vi "Main.vi"(8 "error in":errorcluster, 11 "gRPC Read in":refnum<class "gRPC Read.lvclass">) -> (0 "error out":errorcluster, 3 "gRPC Read out":refnum<class "gRPC Read.lvclass">)   [LabVIEW 2019, in "gRPC Server (scope.proto).lvlib" / "gRPC Read.lvclass"]
doc: "The <b>Queued Message Handler</b> of the Worker that owns this VI."
uses:
  gRPC Read.lvclass
  Initialization Data.ctl
  Response Cases.ctl
  <vilib>/addons/_Workers/Library/Case Label.ctl
  <vilib>/gRPC/LabVIEW gRPC Library/Shared/grpcId.ctl
  gRPC Read.lvclass/gRPC Read.ctl
  rql_Read Incoming Data from Client.ctl
  Generated_server/RPC Messages/w4lvgrpc_ToServer_payload/w4lvgrpc_ToServer_payload.lvclass/w4lvgrpc_ToServer_payload.ctl
  Generated_server/RPC Messages/Get w4lvgrpc_ToServer.vi
  Generated_server/RPC Messages/Get w4lvgrpc_ToServer.vi/2ed25e12-861d-4677-8ead-ace2906b2041.vi
  Generated_server/RPC Messages/FlatToRichw4lvgrpc_ToServer.vi
  <vilib>/gRPC/LabVIEW gRPC Library/Shared/TranslateGrpcError.vi
  Generated_server/RPC Messages/w4lvgrpc_ToServer_payload/Setmsg_1.vi
  Generated_server/RPC Messages/FlatToRichw4lvgrpc_Msg_ToServer_1.vi
  Generated_server/RPC Messages/w4lvgrpc_ToServer_payload/Setmsg_2.vi
  Generated_server/RPC Messages/FlatToRichw4lvgrpc_Msg_ToServer_2.vi
  Generated_server/RPC Messages/w4lvgrpc_ToServer_payload/Setmsg_3.vi
  Generated_server/RPC Messages/FlatToRichw4lvgrpc_Msg_ToServer_3.vi
  Generated_server/RPC Messages/w4lvgrpc_ToServer_payload/Setmsg_4.vi
  Generated_server/RPC Messages/FlatToRichw4lvgrpc_Msg_ToServer_4.vi
  Generated_server/RPC Messages/w4lvgrpc_ToServer_payload/Setmsg_5.vi
  Generated_server/RPC Messages/FlatToRichw4lvgrpc_Msg_ToServer_5.vi
  Generated_server/RPC Messages/w4lvgrpc_ToServer_payload/Setmsg_6.vi
  Generated_server/RPC Messages/FlatToRichw4lvgrpc_Msg_ToServer_6.vi
  Generated_server/RPC Messages/w4lvgrpc_ToServer_payload/Setmsg_7.vi
  Generated_server/RPC Messages/FlatToRichw4lvgrpc_Msg_ToServer_7.vi
  Generated_server/RPC Messages/w4lvgrpc_ToServer_payload/Setmsg_8.vi
  Generated_server/RPC Messages/FlatToRichw4lvgrpc_Msg_ToServer_8.vi
  Generated_server/RPC Messages/w4lvgrpc_ToServer_payload/Setmsg_9.vi
  Generated_server/RPC Messages/FlatToRichw4lvgrpc_Msg_ToServer_9.vi
  Generated_server/RPC Messages/w4lvgrpc_ToServer_payload/GetActiveFieldName.vi
  <vilib>/gRPC/LabVIEW gRPC Library/Server API/Server/Get Server DLL Path.vi
  <vilib>/Utility/error.llb/Error Cluster From Error Code.vi
  Generated_server/RPC Messages/w4lvgrpc_ToServer_payload/w4lvgrpc_ToServer_payload.lvclass
  <vilib>/addons/_Workers/Library/Workers.lvlib
  Generated_server/RPC Service/Session/Session.lvclass
  <vilib>/gRPC/LabVIEW gRPC Library/grpc-lvsupport-release.lvlib
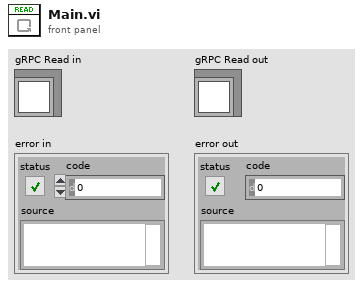
[diagram p1: front panel]
types:
  T1 = typedef "gRPC Server (scope.proto).lvlib/gRPC Read.lvclass/Initialization Data.ctl" = cluster{"Response Cases":T2, "gRPC ID":T4}
  T2 = typedef "gRPC Server (scope.proto).lvlib/gRPC Read.lvclass/Response Cases.ctl" = cluster{"Receive Incoming Data":T3, "Connection Lost":T3, "New Connection":T3}
  T3 = typedef "Workers.lvlib/Case Label.ctl" = string
  T4 = typedef "grpc-lvsupport-release.lvlib/grpcId.ctl" = u64
  T5 = typedef "gRPC Server (scope.proto).lvlib/gRPC Read.lvclass/rql_Read Incoming Data from Client.ctl" = cluster{"Placeholder":string}
  T6 = typedef "Generated_server.lvlib/w4lvgrpc_ToServer.ctl" = cluster{"w4lvgrpc_ToServer_payload":refnum<class "w4lvgrpc_ToServer_payload.lvclass">}
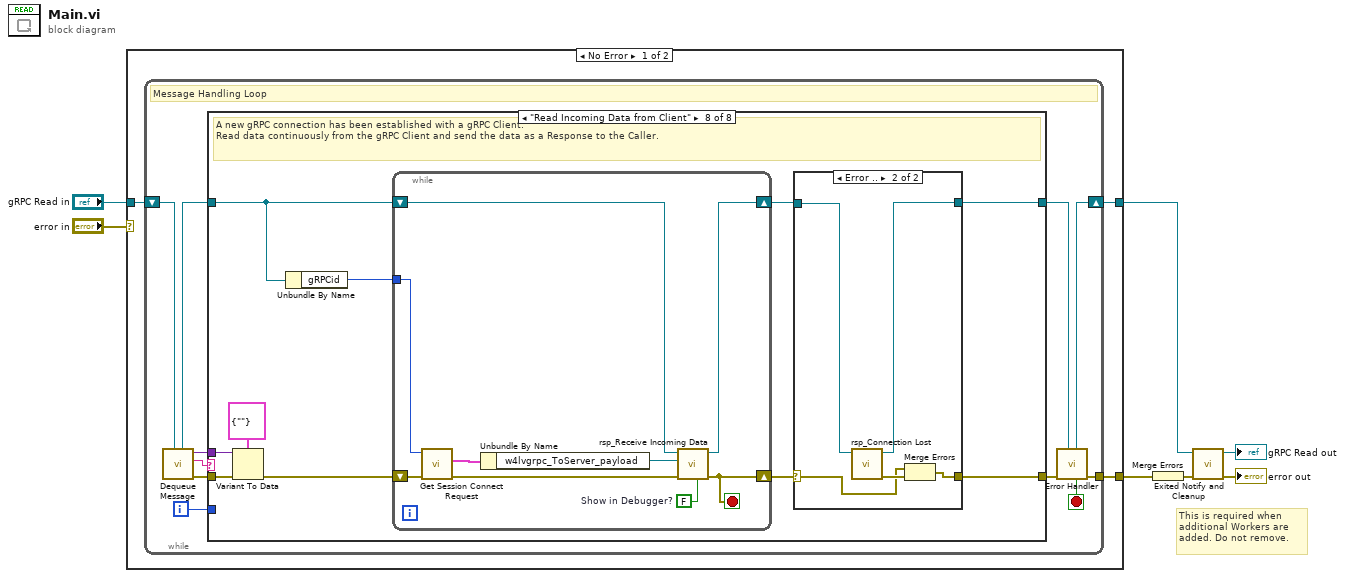
[diagram p0: block diagram]
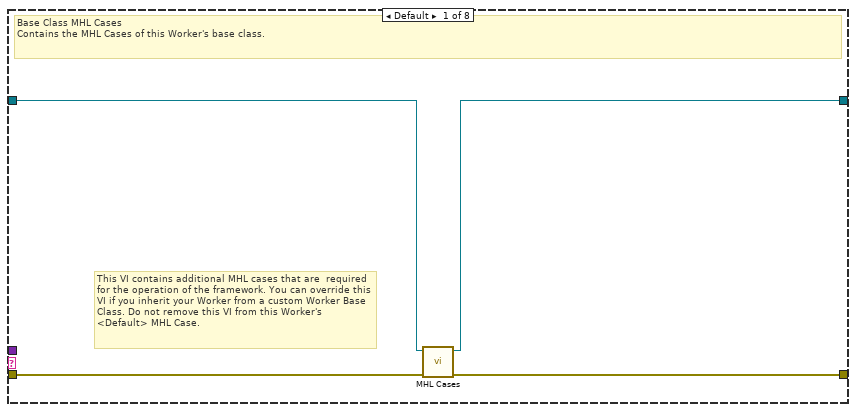
[diagram p2: hidden frame]
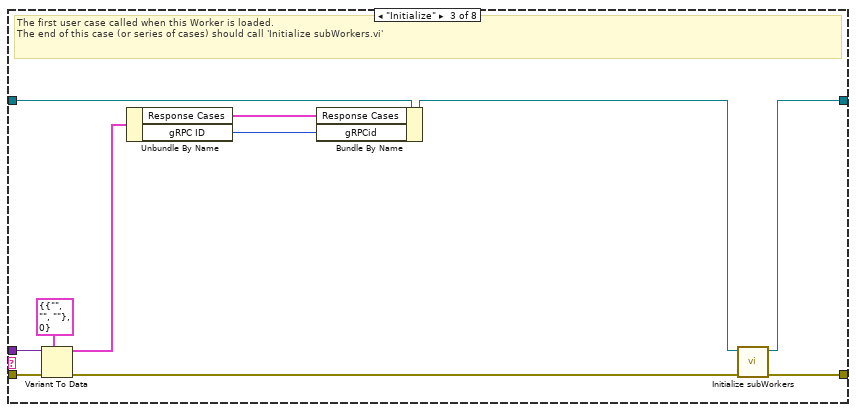
[diagram p4: hidden frame]
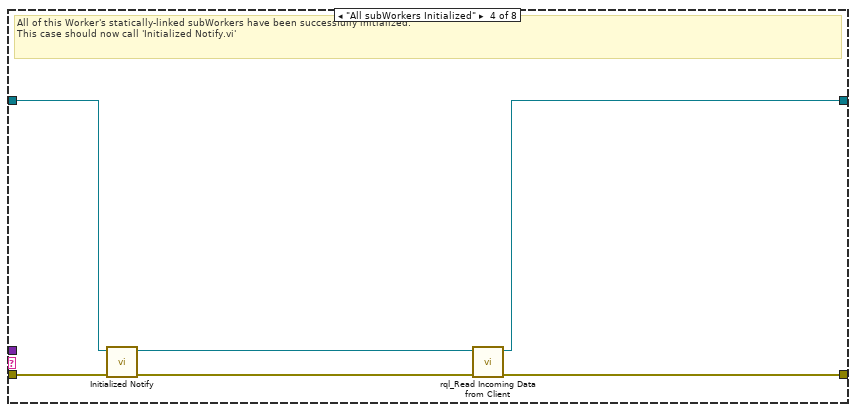
[diagram p5: hidden frame]
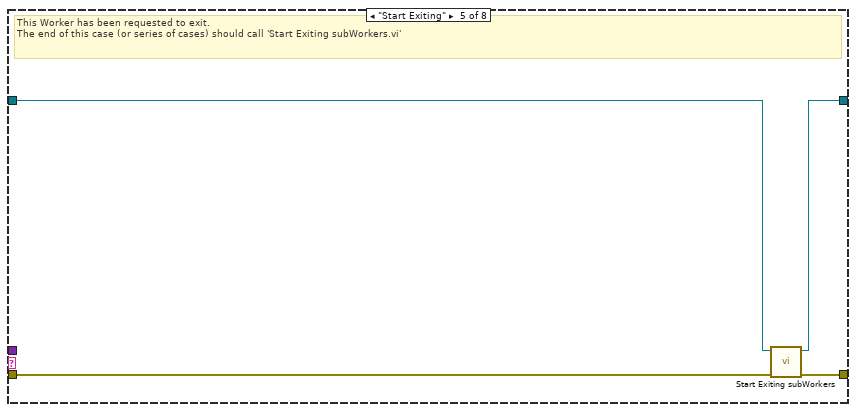
[diagram p6: hidden frame]
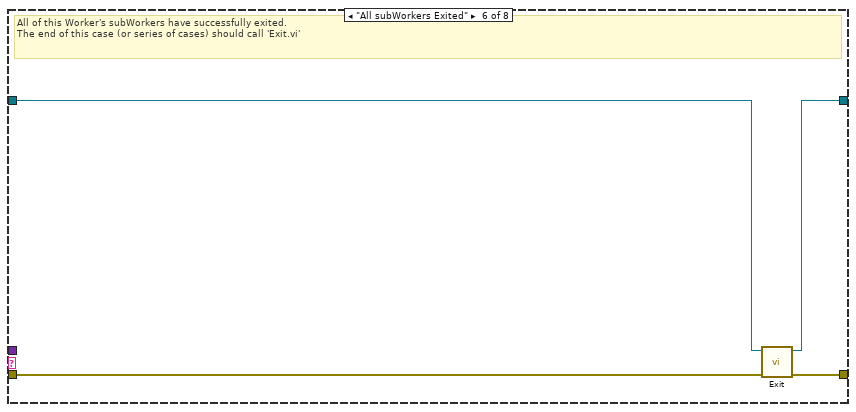
[diagram p7: hidden frame]
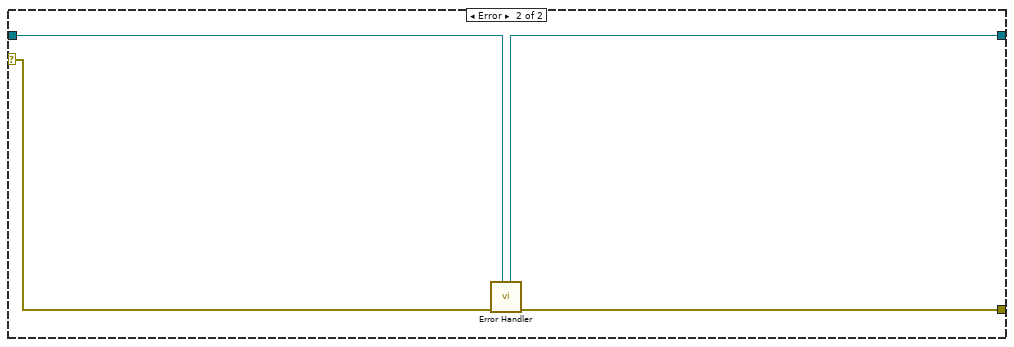
[diagram p10: hidden frame]
diagram:
  # "This is required when additional Workers are added. Do not remove."
  n1 = case shown="No Error" "error in" {
    tunnel: [w10 w83] -> w6
    tunnel: [w9 w82] -> w7
    selector: "error in" -> [_ w84]
    tunnel: "gRPC Read in" -> [w8 w81]
    frame No Error {
      n2 = while {
        shift-right: [w19] -> w9
        shift-left: w8 -> [w21]
        tunnel: [w20] -> w10
        i -> [w12]
        stop <- w13 stop-if-true
        # "Message Handling Loop"
        n3 = call-dynamic "Dequeue Message.vi"("Worker"=w21) -> ("error out"=w18:errorcluster, "Case out"=w14:string, "Data out"=w11:variant, "Worker out"=w16:refnum<class "gRPC Read.lvclass">)  [unwired: 6 in, 1 out]
        n4 = case "Worker MHL Case Structure (DO NOT CHANGE LABEL NAME)" shown="\"Read Incoming Data from Client\"" w14 {
          tunnel: w18 -> [w25 w26 w36 w44 w45 w52 w54 w64]
          tunnel: [w24 w26 w38 w41 w48 w51 w54 w58] -> w17
          tunnel: w16 -> [w23 w27 w35 w42 w46 w50 w53 w56]
          tunnel: [w22 w27 w37 w39 w47 w49 w53 w57] -> w15
          tunnel: w12 -> [_ _ _ _ _ _ _ _]
          tunnel: w11 -> [_ _ w33 _ _ _ _ w62]
          frame Default {
            # "This VI contains additional MHL cases that are  required for the operation of the framework. You can override this VI if you inherit your Worker from a custom Worker Base Class. Do not remove this VI from this Worker's <Default> MHL Case."
            # "Base Class MHL Cases\nContains the MHL Cases of this Worker's base class."
            n5 = call-dynamic "MHL Cases.vi"("error in"=w25, "Worker in"=w23) -> ("error out"=w24:errorcluster, "Worker out"=w22:refnum<class "gRPC Read.lvclass">)  [unwired: 8 in]
          }
          frame "------------ FRAMEWORK CASES -----------" {
            # "Start of Workers Framework Cases"
          }
          frame "Initialize" {
            # "The first user case called when this Worker is loaded.\nThe end of this case (or series of cases) should call 'Initialize subWorkers.vi'"
            n6 = Variant To Data(error in=w36, type=T1 {"Response Cases"={"Receive Incoming Data"="", "Connection Lost"="", "New Connection"=""}, "gRPC ID"=0} ("Cluster"), Variant=w33) -> (data=w31:T1, error out=w34:errorcluster)
            n7 = Unbundle By Name(w31) -> ("Response Cases"=w30:T2, "gRPC ID"=w28:T4)
            n8 = Bundle By Name(cluster=w35, "Response Cases"=w30, "gRPCid"=w28) -> (w32:refnum<class "gRPC Read.lvclass">)
            n9 = call-dynamic "Initialize subWorkers.vi"("error in"=w34, "Worker"=w32) -> ("error out"=w38:errorcluster, "dup Worker out"=w37:refnum<class "gRPC Read.lvclass">)  [unwired: 8 in]
          }
          frame "All subWorkers Initialized" {
            # "All of this Worker's statically-linked subWorkers have been successfully initialized.\nThis case should now call 'Initialized Notify.vi'"
            n10 = call-dynamic "Initialized Notify.vi"("error in"=w44, "Worker"=w42) -> ("error out"=w43:errorcluster, "dup Worker out"=w40:refnum<class "gRPC Read.lvclass">)  [unwired: 8 in]
            n11 = call "rql_Read Incoming Data from Client.vi"("error in"=w43, "gRPC Read in"=w40) -> ("error out"=w41:errorcluster, "dup gRPC Read out"=w39:refnum<class "gRPC Read.lvclass">)  [unwired: 8 in]
          }
          frame "Start Exiting" {
            # "This Worker has been requested to exit. \nThe end of this case (or series of cases) should call 'Start Exiting subWorkers.vi'"
            n12 = call-dynamic "Start Exiting subWorkers.vi"("error_in"=w45, "Worker"=w46) -> ("error out"=w48:errorcluster, "dup Worker out"=w47:refnum<class "gRPC Read.lvclass">)  [unwired: 8 in]
          }
          frame "All subWorkers Exited" {
            # "All of this Worker's subWorkers have successfully exited. \nThe end of this case (or series of cases) should call 'Exit.vi'"
            n13 = call-dynamic "Exit.vi"("error_in"=w52, "Worker"=w50) -> ("error out"=w51:errorcluster, "dup Worker out"=w49:refnum<class "gRPC Read.lvclass">)  [unwired: 8 in]
          }
          frame "------------- LOCAL API CASES -------------" {
            # "Start of Workers Local API Cases"
          }
          frame "Read Incoming Data from Client" {
            # "A new gRPC connection has been established with a gRPC Client.\nRead data continuously from the gRPC Client and send the data as a Response to the Caller."
            n14 = Variant To Data(error in=w64, type=T5 {"Placeholder"=""} ("Data"), Variant=w62) -> (error out=w59:errorcluster)  [unwired: 1 out]
            n15 = Unbundle By Name(w56) -> ("gRPCid"=w55:T4)
            n16 = while {
              shift-right: [w76] -> w60
              shift-left: w59 -> [w74]
              shift-right: [w77] -> w61
              shift-left: w56 -> [w80]
              tunnel: w55 -> [w75]
              stop <- w76 stop-if-true
              w78 = FALSE  # Show in Debugger?
              n17 = call "Get Session Connect Request.vi"("error in (no error)"=w74, "gRPCid"=w75) -> ("error out"=w73:errorcluster, "Message Data"=w72:T6)  [unwired: 7 in, 1 out]
              n18 = Unbundle By Name(w72) -> ("w4lvgrpc_ToServer_payload"=w79:refnum<class "w4lvgrpc_ToServer_payload.lvclass">)
              n19 = call "rsp_Receive Incoming Data.vi"("Show in Debugger?"=w78, "error in"=w73, "Data in"=w79, "gRPC Read in"=w80) -> ("error out"=w76:errorcluster, "dup gRPC Read out"=w77:refnum<class "gRPC Read.lvclass">)  [unwired: 6 in]
            }
            n20 = case shown="Error .." w60 {
              selector: w60 -> [w65 w68]
              tunnel: [w65 w69] -> w58
              tunnel: [w66 w70] -> w57
              tunnel: w61 -> [w66 w67]
              frame No Error {
              }
              frame Error {
                n21 = call "rsp_Connection Lost.vi"("gRPC Read in"=w67) -> ("error out"=w71:errorcluster, "dup gRPC Read out"=w70:refnum<class "gRPC Read.lvclass">)  [unwired: 9 in]
                n22 = Merge Errors(w68, w71) -> (w69:errorcluster)
              }
            }
          }
        }
        n23 = call-dynamic "Error Handler.vi"("Worker"=w15, "error_in"=w17) -> ("error out"=w20:errorcluster, "Stop Loop"=w13:bool, "Worker out"=w19:refnum<class "gRPC Read.lvclass">)  [unwired: 7 in]
      }
    }
    frame Error {
      n24 = call-dynamic "Error Handler.vi"("Worker"=w81, "error_in"=w84) -> ("error out"=w83:errorcluster, "Worker out"=w82:refnum<class "gRPC Read.lvclass">)  [unwired: 7 in, 1 out]
    }
  }
  n25 = Merge Errors(w6) -> (w3:errorcluster)
  n26 = call-dynamic "Exited Notify and Cleanup.vi"("error_in"=w3, "Worker"=w7) -> ("error out"=→"error out":errorcluster, "dup Worker out"=→"gRPC Read out":refnum<class "gRPC Read.lvclass">)  [unwired: 8 in]
